vi "SlowLogger_SetMaxLogSpeed.vi"(8 "error in (no error)":errorcluster, 10 "Max Log Speed [Delta Time] (seconds)":dbl=10.0, 11 "SlowLogger in":refnum<class "SlowLogger.lvclass">) -> (0 "error out":errorcluster, 3 "SlowLogger out":refnum<class "SlowLogger.lvclass">)   [LabVIEW 2018, in "SlowLogger.lvclass"]
uses:
  SlowLogger.lvclass
  SlowLogger.lvclass/SlowLogger.ctl
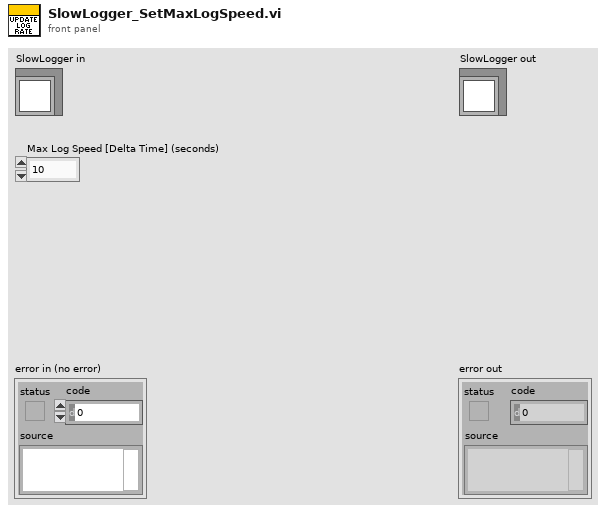
[diagram p1: front panel]
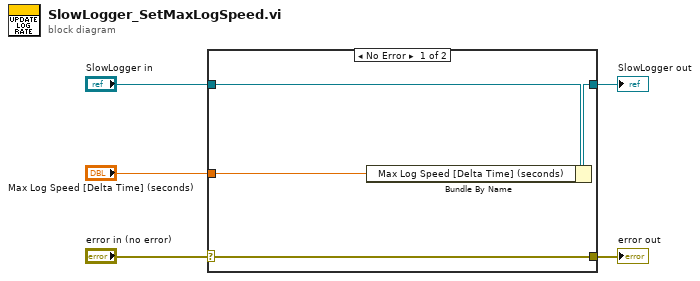
[diagram p0: block diagram]
diagram:
  n1 = case shown="No Error" "error in (no error)" {
    selector: "error in (no error)" -> [w9 w10]
    tunnel: [w9 w10] -> w4
    tunnel: [w7 w11] -> w2
    tunnel: "SlowLogger in" -> [w8 w11]
    tunnel: "Max Log Speed [Delta Time] (seconds)" -> [w6 _]
    frame No Error {
      n2 = Bundle By Name(cluster=w8, "Max Log Speed [Delta Time] (seconds)"=w6) -> (w7:refnum<class "SlowLogger.lvclass">)
    }
    frame Error {
    }
  }
  "error out" <- w4
  "SlowLogger out" <- w2
